vi "Scan Module.vi"(7 "Slice pattern":T1={"repitition"=14, "thick slice (um)"=500.0, "thin slice (um)"=100.0} {"thin slice (um)" format="%#_13g"; "thick slice (um)" format="%#_13g"}, 8 "Error In":errorcluster, 9 "System Parameters":T2={"Vibratome"={"Z Bottom [mm]"=0.0, "Pre Cut Dwell [s]"=1.0, "Blade Frequency [RPM]"=3000, "Slice Speed [mm/s]"=0.1, "Post Cut Dwell [s]"=4.0, "Ramp Time [s]"=0.5, "Start X [mm]"=80.5, "Start Y [mm]"=72.0, "Slice Length [mm]"=15.0, "Slice Axis"=enum."X Axis", "Controller VISA Ref"="COM3"}, "Table Stages"={"X Stage"={"Position"=0.0, "Is.Enabled?"=FALSE, "Is.Connected?"=FALSE, "Device SN"="45875688", "AccelerationMaximum"=50.0, "VelocityMaximum"=50.0, "Acceleration"=20.0, "Velocity"=20.0, "waitTimeout (ms)"=1000000, "Model"=enum."Thorlabs LTS", "Is.Homed?"=FALSE}, "Y Stage"={"Position"=0.0, "Is.Enabled?"=FALSE, "Is.Connected?"=FALSE, "Device SN"="45875512", "AccelerationMaximum"=50.0, "VelocityMaximum"=50.0, "Acceleration"=20.0, "Velocity"=20.0, "waitTimeout (ms)"=1000000, "Model"=enum."Thorlabs LTS", "Is.Homed?"=FALSE}, "Z Stage"={"Position"=0.0, "Is.Enabled?"=FALSE, "Is.Connected?"=FALSE, "Device SN"="49872414", "AccelerationMaximum"=50.0, "VelocityMaximum"=50.0, "Acceleration"=20.0, "Velocity"=20.0, "waitTimeout (ms)"=100000, "Model"=enum."Thorlabs MLJ", "Is.Homed?"=FALSE}}}, 10 "Mosaic Parameters":T5={"Overlap Options"={"Overlap Type"=enum."No Overlap", "Percent Overlap"=0, "Justify"=enum."Start"}, "Mosaic Range"={"X Axis"={"Start [mm]"=10.0, "Steps [pts]"=0, "End [mm]"=28.0}, "Y Axis"={"Start [mm]"=45.0, "Steps [pts]"=0, "End [mm]"=63.0}}, "Scan Pattern"=enum."Uni-directional", "Number of slices"=1} {"Overlap Options"."Percent Overlap" max=50}, 11 "Imaging Parameters":T6={"Save Path"=path "E:/Jiarui/1217test", "# Cscan"=1, "ROI Parameters"={"ROI (mm)"={"X (mm)"=1.0, "Y (mm)"=1.0}, "Shift (mm)"={"Xshift (mm)"=0.0, "Yshift (mm)"=0.0}}, "Scan Parameters"={"# Scan"={"#Ascan"=400, "#Bscan"=400}, "# Rpt"={"#ARpt"=1, "#BRpt"=1}, "Aline Rate"=2, "# Extra"={"# ARpt_extra"=5, "#Brtn_extra"=80}}, "Objective"=0, "Image Index"=0} {"Objective" items=["5X LKM05", "10X LKM10", "20X LKM20", "10X LSM02"]; "Scan Parameters"."Aline Rate" items=["76 KHz", "146 KHz", "76 KHz", "28 KHz", "10 KHz"]}) -> (0 "Error Out":errorcluster, 3 "Finished?":bool)   [LabVIEW 2017]
uses:
  Controls/Go Scan Actions.ctl
  Controls/System Parameters.ctl
  Hardware/Table Stage/Controls/Translation Stage Cluster.ctl
  Controls/Translation Stage Types.ctl
  Controls/FGV Actions.ctl
  Controls/ScanType.ctl
  Hardware/Table Stage/Controls/Motion Translation Module Control.ctl
  Controls/Set Get Controls.ctl
panel:
  out "Waveform Chart":dbl(graph)
  out "Current State":T7
  out "Current Position":cluster{"X":dbl, "Y":dbl}
  out "XY Graph":cluster{"X":dbl, "Y":dbl}[](graph)
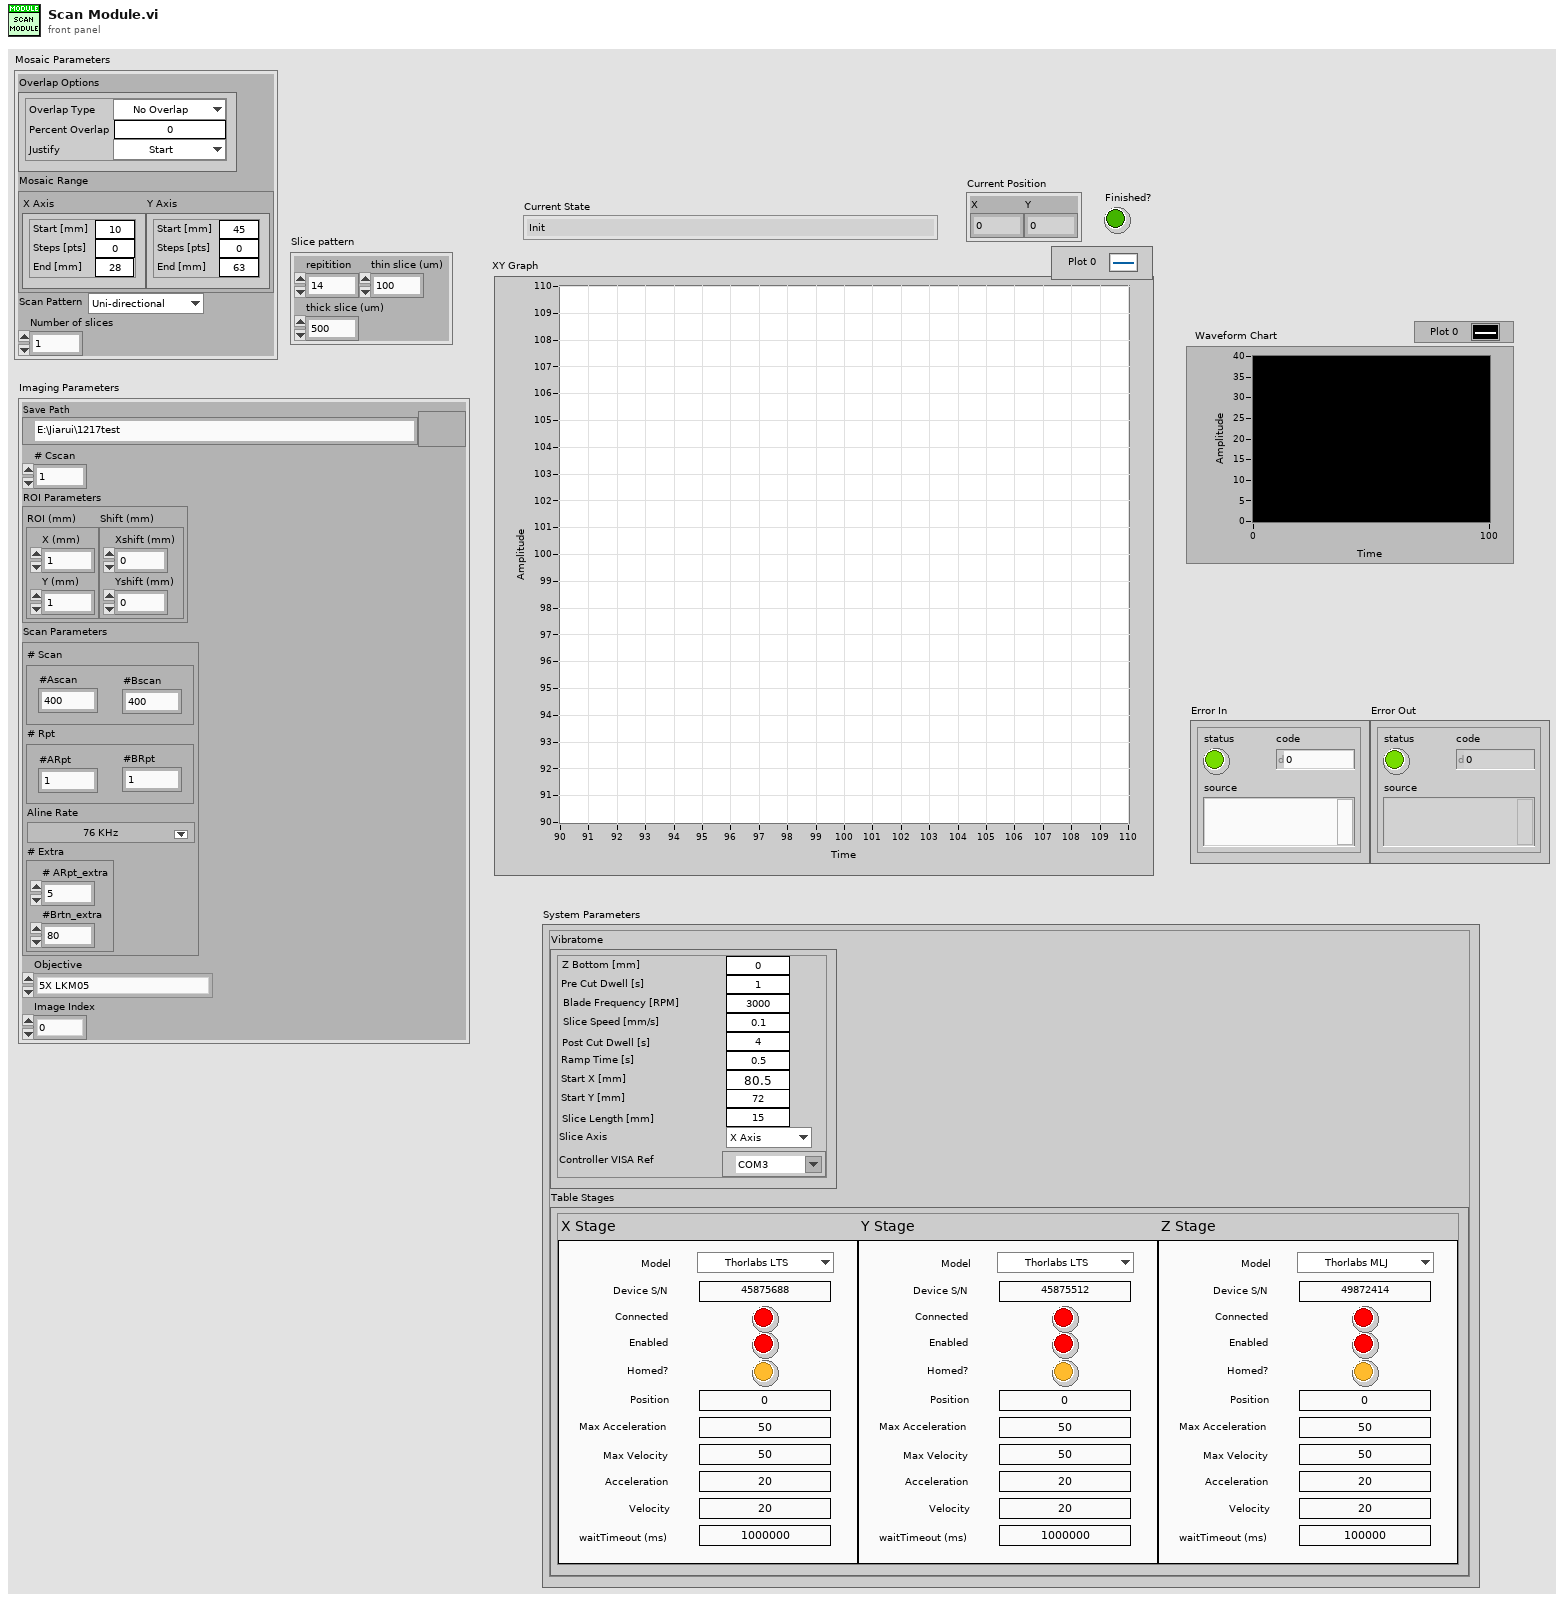
[diagram p1: front panel]
types:
  T1 = cluster{"repitition":i32, "thick slice (um)":dbl, "thin slice (um)":dbl}
  T2 = typedef "System Parameters.ctl" = cluster{"Vibratome":cluster{"Z Bottom [mm]":dbl, "Pre Cut Dwell [s]":dbl, "Blade Frequency [RPM]":u16, "Slice Speed [mm/s]":dbl, "Post Cut Dwell [s]":dbl, "Ramp Time [s]":dbl, "Start X [mm]":dbl, "Start Y [mm]":dbl, "Slice Length [mm]":dbl, "Slice Axis":enum16{"X Axis", "Y Axis", "Z Axis"}, "Controller VISA Ref":refnum<visa-resource-name>}, "Table Stages":cluster{"X Stage":T3, "Y Stage":T3, "Z Stage":T3}}
  T3 = typedef "Translation Stage Cluster.ctl" = cluster{"Position":dbl, "Is.Enabled?":bool, "Is.Connected?":bool, "Device SN":string, "AccelerationMaximum":dbl, "VelocityMaximum":dbl, "Acceleration":dbl, "Velocity":dbl, "waitTimeout (ms)":i32, "Model":T4, "Is.Homed?":bool}
  T4 = typedef "Translation Stage Types.ctl" = enum16{"None", "Thorlabs LTS", "Thorlabs MLJ"}
  T5 = cluster{"Overlap Options":cluster{"Overlap Type":enum16{"No Overlap", "X Only", "Y Only", "X and Y"}, "Percent Overlap":u8, "Justify":enum16{"Start", "Center", "End"}}, "Mosaic Range":cluster{"X Axis":cluster{"Start [mm]":dbl, "Steps [pts]":u16, "End [mm]":dbl}, "Y Axis":cluster{"Start [mm]":dbl, "Steps [pts]":u16, "End [mm]":dbl}}, "Scan Pattern":enum16{"Uni-directional", "Bi-Directional", "Spiral Out", "Spiral In"}, "Number of slices":i16}
  T6 = cluster{"Save Path":path, "# Cscan":i32, "ROI Parameters":cluster{"ROI (mm)":cluster{"X (mm)":sgl, "Y (mm)":sgl}, "Shift (mm)":cluster{"Xshift (mm)":sgl, "Yshift (mm)":sgl}}, "Scan Parameters":cluster{"# Scan":cluster{"#Ascan":i32, "#Bscan":i32}, "# Rpt":cluster{"#ARpt":i32, "#BRpt":i32}, "Aline Rate":u16, "# Extra":cluster{"# ARpt_extra":i32, "#Brtn_extra":i32}}, "Objective":u16, "Image Index":i16}
  T7 = typedef "Go Scan Actions.ctl" = enum16{"Init", "Init Scan Head", "Init Table Stage", "Init Vibratome", "Generate Mosaic", "Go Image Home", "Go Mosaic", "Acquire Image", "Go Vibratome", "Slice", "Finished"}
  T8 = cluster{"Start [mm]":dbl, "Steps [pts]":u16, "End [mm]":dbl}
  T9 = enum16{"Uni-directional", "Bi-Directional", "Spiral Out", "Spiral In"}
  T10 = cluster{"Overlap Type":enum16{"No Overlap", "X Only", "Y Only", "X and Y"}, "Percent Overlap":u8, "Justify":enum16{"Start", "Center", "End"}}
  T11 = typedef "FGV Actions.ctl" = enum16{"Init", "Set", "Get", "Clear"}
  T12 = typedef "ScanType.ctl" = enum16{"Single Frame", "Continuous Frame", "ROI Line", "Vibratome", "Mosaic", "Mosaic + Slice"}
  T13 = enum16{"Init", "Configure", "Configure Data", "Generate Scan Pattern", "Start Acquire Raw", "Start Acquire Data", "Acquire RAW", "Acquire Data", "Stop Acquire", "Uninit"}
  T14 = enum16{"Create", "Enqueue", "Dequeue", "Release"}
  T15 = typedef "Set Get Controls.ctl" = enum16{"Set", "Get"}
  T16 = typedef "Motion Translation Module Control.ctl" = enum16{"Init", "Home", "Status", "Velocity/Accel", "Position", "Jog", "Stop", "Uninit", "Enable", "Disable"}
  T17 = cluster{"Objective":u16, "Aline Rate":u16, "# Cscan":i32, "ROI Parameters":cluster{"ROI (mm)":cluster{"X (mm)":sgl, "Y (mm)":sgl}, "Shift (mm)":cluster{"Xshift (mm)":sgl, "Yshift (mm)":sgl}}}
  T18 = cluster{"Image Index":i16, "Slice Index":i16, "#Cscan":i32, "nAT per B":i32, "nA per B":i32, "Brtn_extra/2":i32}
  T19 = cluster{"# Scan":cluster{"#Ascan":i32, "#Bscan":i32}, "# Rpt":cluster{"#ARpt":i32, "#BRpt":i32}, "Aline Rate":u16, "# Extra":cluster{"# ARpt_extra":i32, "#Brtn_extra":i32}}
  T20 = cluster{"ROI (mm)":cluster{"X (mm)":sgl, "Y (mm)":sgl}, "Shift (mm)":cluster{"Xshift (mm)":sgl, "Yshift (mm)":sgl}}
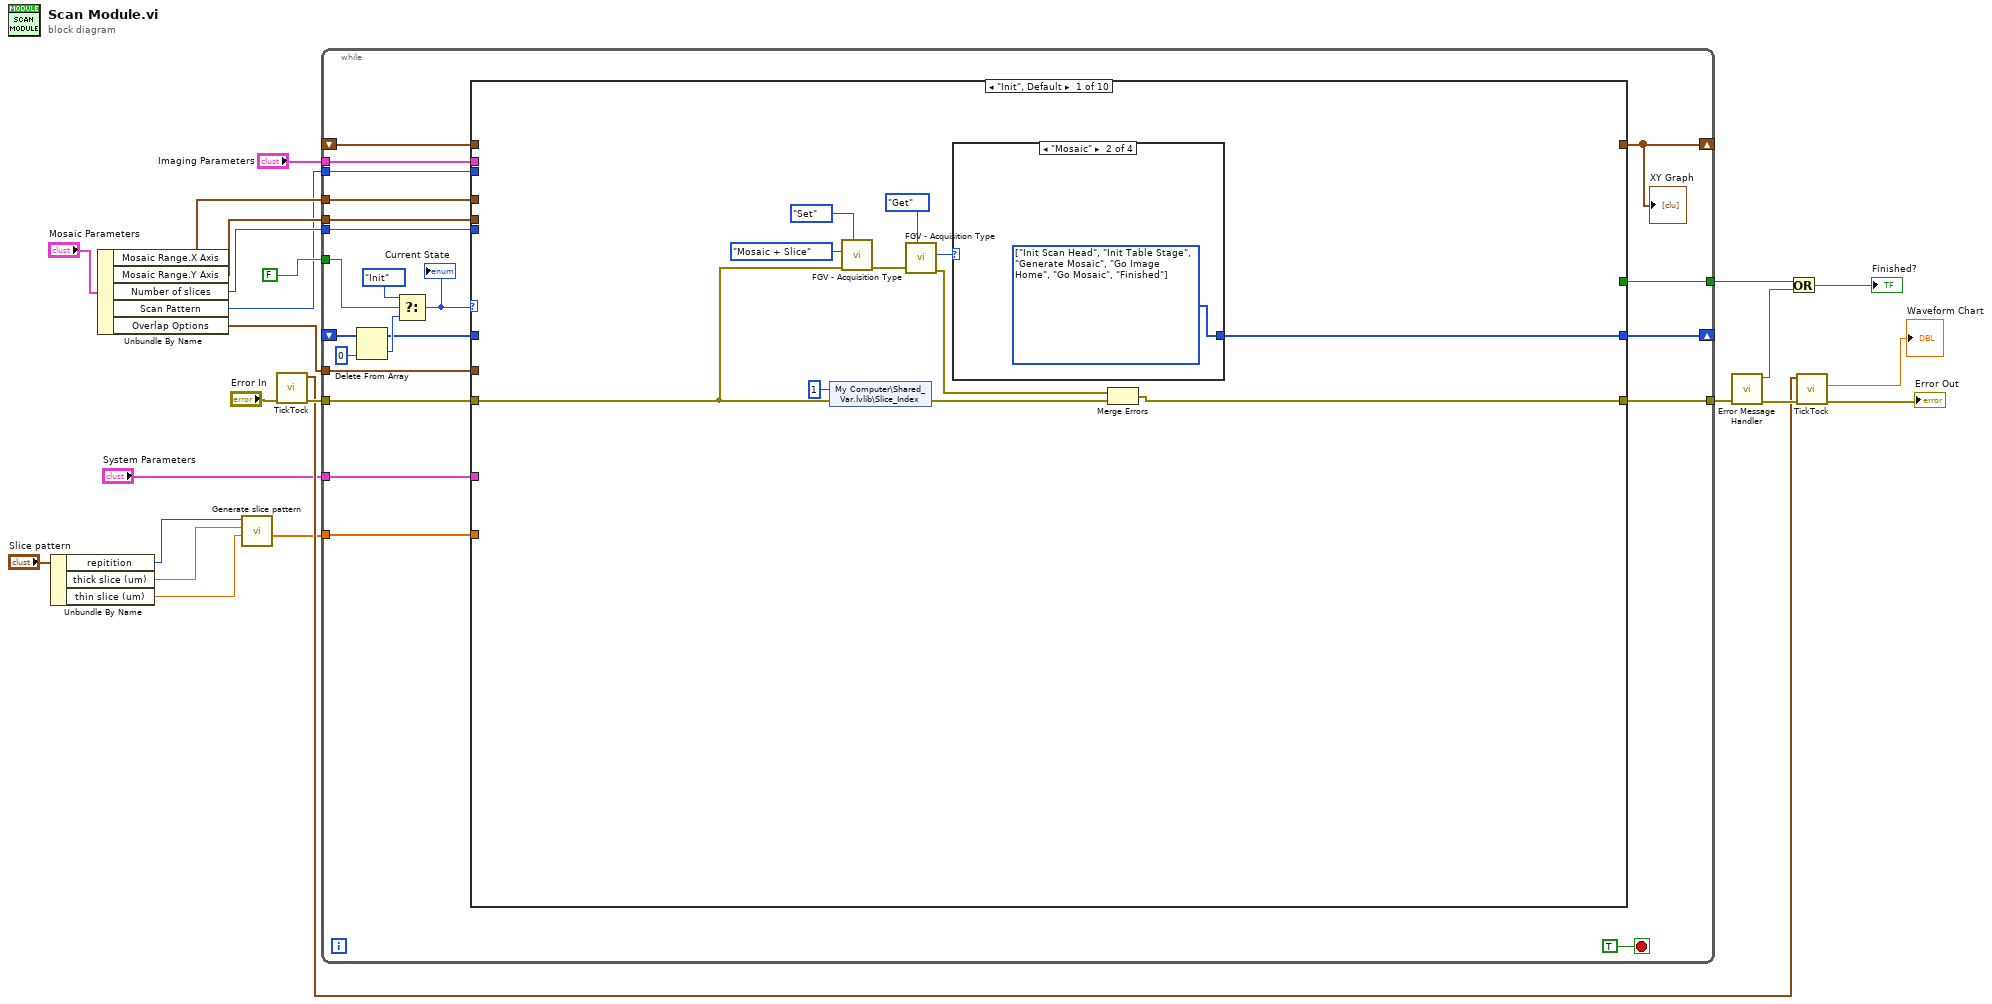
[diagram p0: block diagram]
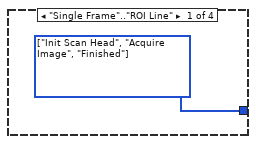
[diagram p2: hidden frame]
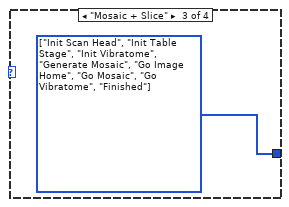
[diagram p3: hidden frame]
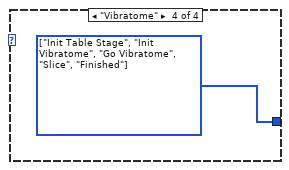
[diagram p4: hidden frame]
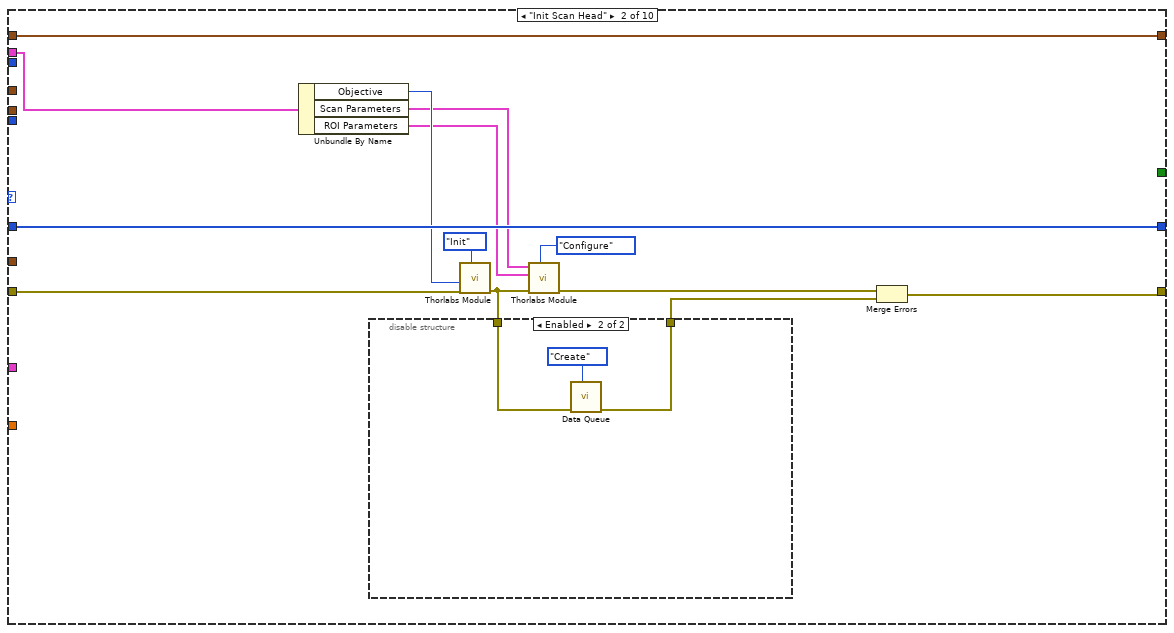
[diagram p5: hidden frame]
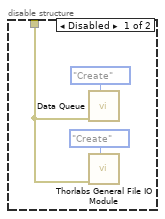
[diagram p6: hidden frame]
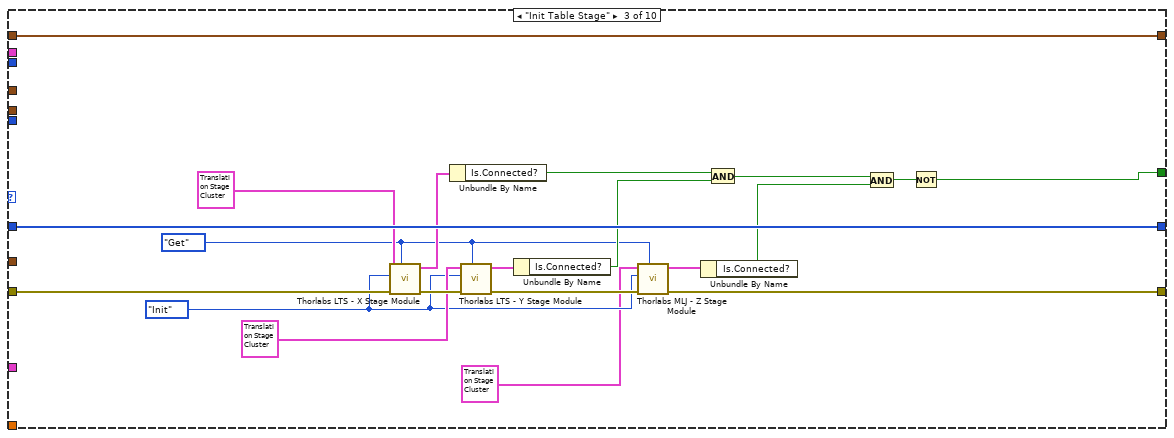
[diagram p7: hidden frame]
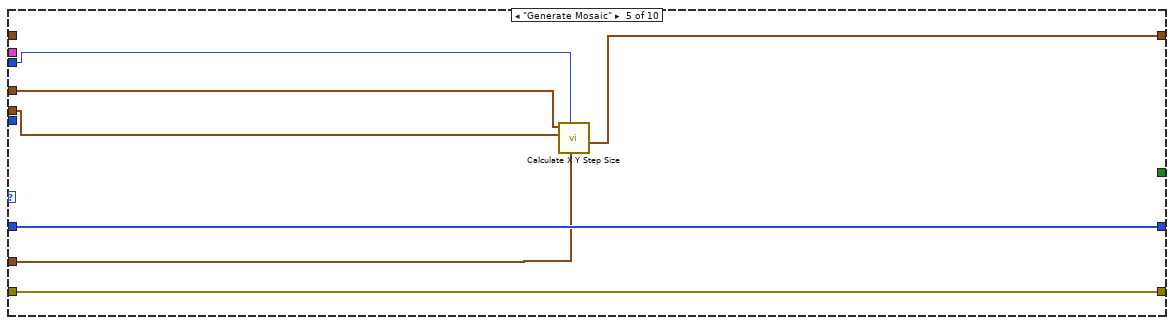
[diagram p9: hidden frame]
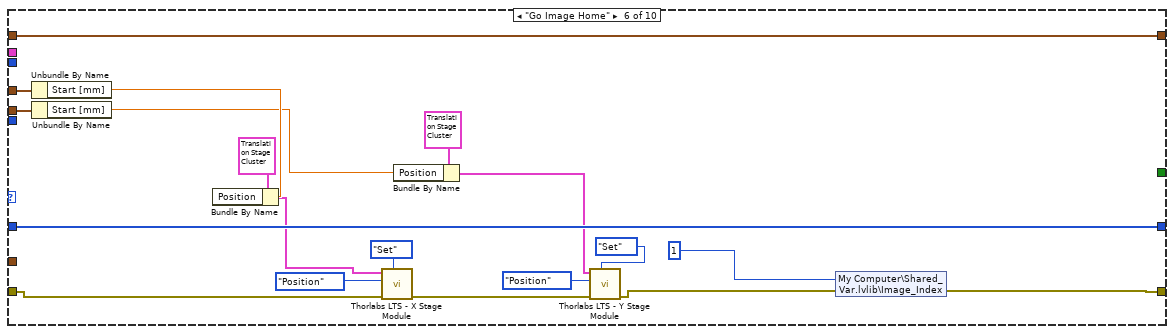
[diagram p10: hidden frame]
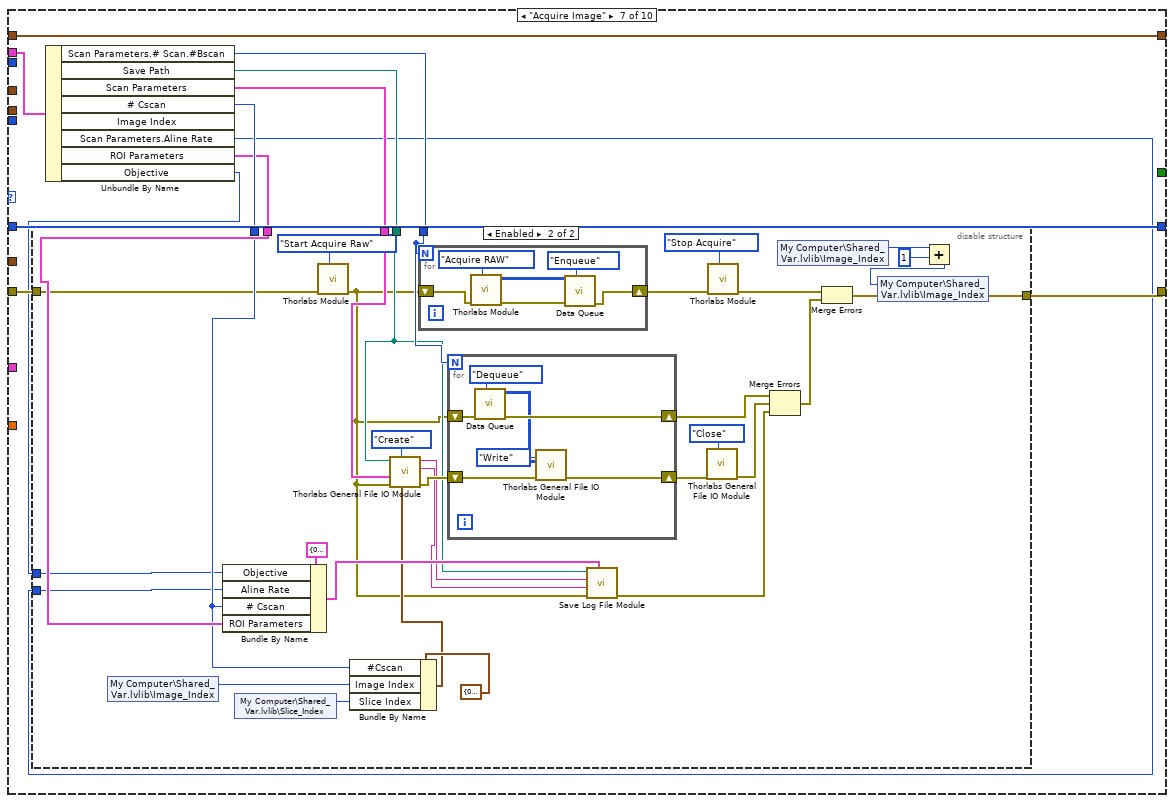
[diagram p11: hidden frame]
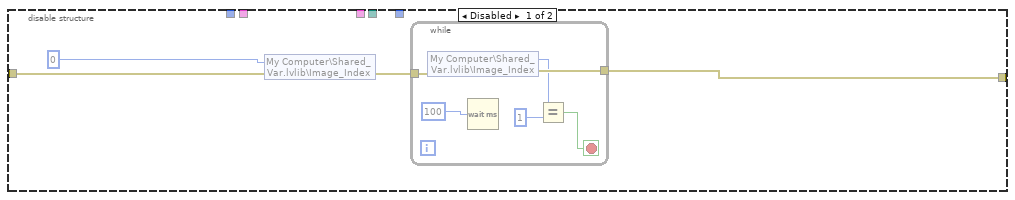
[diagram p12: hidden frame]
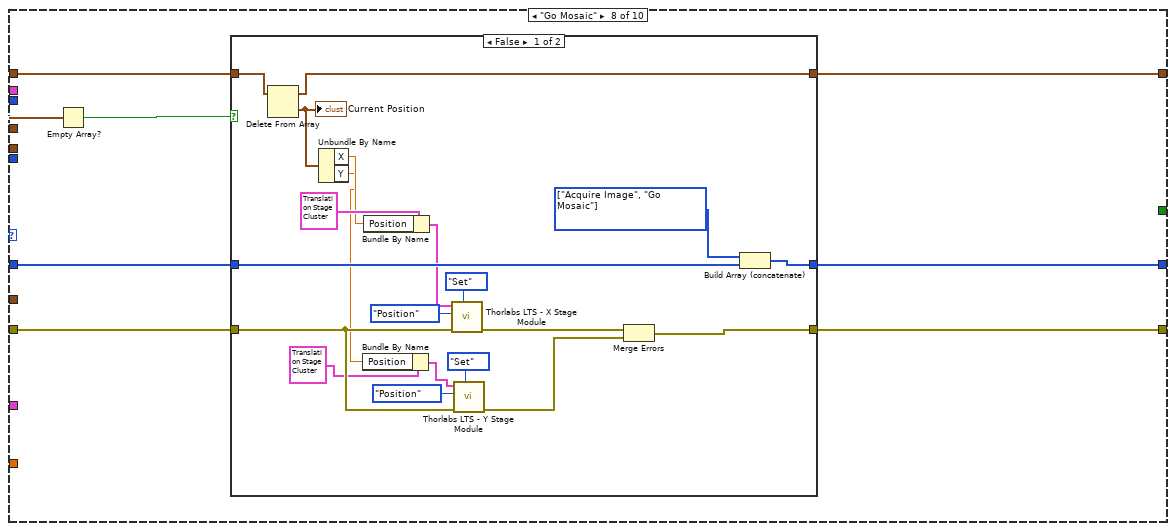
[diagram p13: hidden frame]
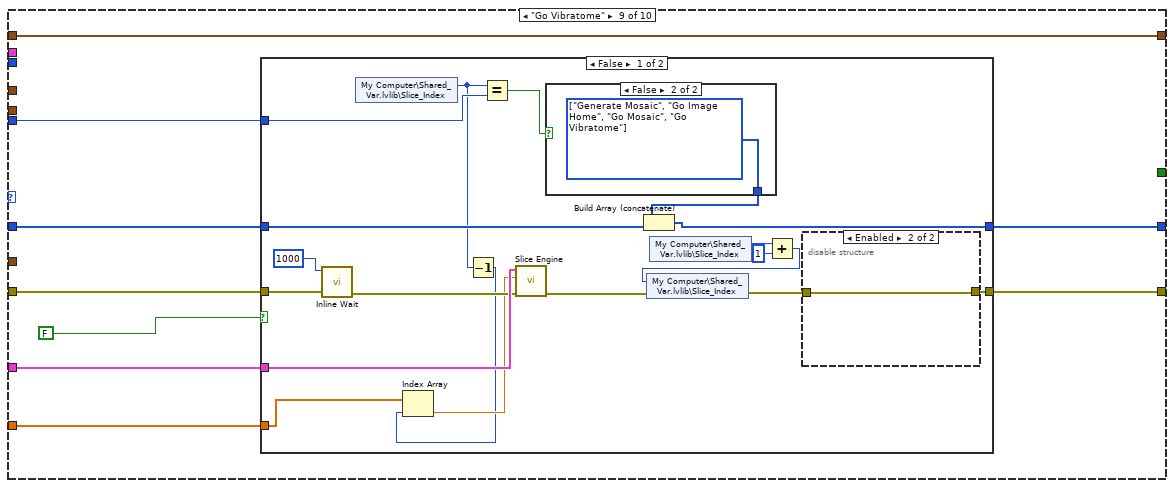
[diagram p15: hidden frame]
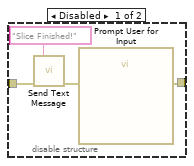
[diagram p16: hidden frame]
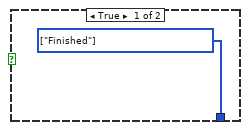
[diagram p17: hidden frame]
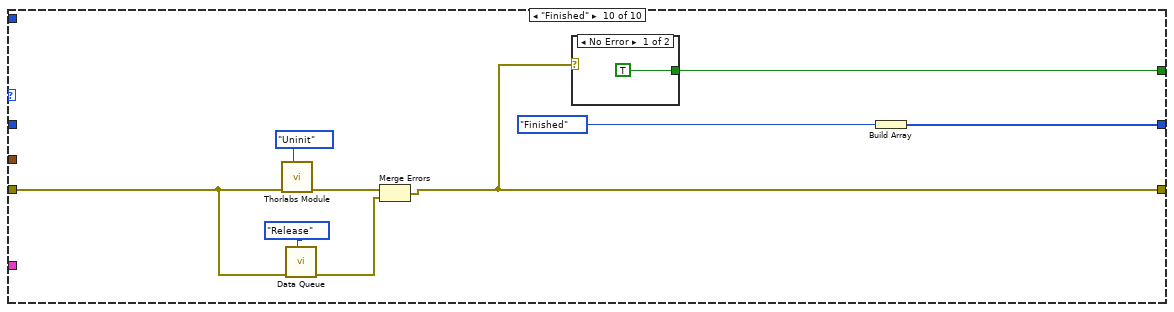
[diagram p19: hidden frame]
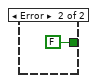
[diagram p20: hidden frame]
diagram:
  n1 = Unbundle By Name("Slice pattern") -> ("repitition"=w3:i32, "thick slice (um)"=w2:dbl, "thin slice (um)"=w1:dbl)
  n2 = Unbundle By Name("Mosaic Parameters") -> ("Mosaic Range.X Axis"=w12:T8, "Mosaic Range.Y Axis"=w11:T8, "Number of slices"=w9:i16, "Scan Pattern"=w7:T9, "Overlap Options"=w8:T10)
  n3 = call "Generate slice pattern.vi"("thin slice (um)"=w1, "thick slice (um)"=w2, "repitition"=w3) -> ("Array"=w5:dbl[])  [unwired: 8 in]
  n4 = call "TickTock.vi"("Error In"="Error In") -> ("Error Out"=w17:errorcluster, "Current Time (Out)"=w15:timestamp)  [unwired: 8 in, 1 out]
  n5 = while {
    shift-right: [w43] -> _
    shift-left: _ -> [w42]
    tunnel: FALSE ("Init") -> [w45]
    shift-right: [w38] -> _
    shift-left: _ -> [w39]
    tunnel: [w37] -> w23
    tunnel: w17 -> [w35]
    tunnel: [w34] -> w22
    tunnel: w12 -> [w32]
    tunnel: w11 -> [w31]
    tunnel: "Imaging Parameters" -> [w30]
    tunnel: w9 -> [w29]
    tunnel: w8 -> [w28]
    tunnel: w7 -> [w27]
    tunnel: "System Parameters" -> [w26]
    tunnel: w5 -> [w25]
    stop <- TRUE stop-if-true
    n6 = Delete From Array(array=w42, index=0) -> (deleted portion=w41:T7, array with subset deleted=w40:T7[])  [unwired: 1 in]
    n7 = Select(t=Go_Scan_Actions."Init", s=w45, f=w41) -> (s? t:f=w44:T7)
    "Current State" <- w44
    n8 = case shown="\"Init\", Default" w44 {
      tunnel: [w55 w73 w99 w102 w110 w128 w140 w201 w234 w273] -> w43
      tunnel: w40 -> [_ w73 w99 w102 w110 w128 w140 w202 w235 _]
      tunnel: [_ w74 w100 w103 w108 w129 w141 w205 w237 _] -> w38
      tunnel: w39 -> [_ w74 w100 w103 _ w129 w141 w204 w237 _]
      tunnel: [_ _ w94 _ _ _ _ _ _ w272] -> w37
      tunnel: w35 -> [w49 w71 w98 w101 w109 w124 w139 w200 w233 w271]
      tunnel: [w50 w64 w88 w101 w109 w127 w138 w199 w232 w266] -> w34
      tunnel: w32 -> [_ _ _ _ w107 w125 _ _ _ _]
      tunnel: w31 -> [_ _ _ _ w106 w115 _ _ _ _]
      tunnel: w30 -> [_ w72 _ _ _ _ w137 _ _ _]
      tunnel: w29 -> [_ _ _ _ _ _ _ _ w231 _]
      tunnel: w28 -> [_ _ _ _ w105 _ _ _ _ _]
      tunnel: w27 -> [_ _ _ _ w104 _ _ _ _ _]
      tunnel: w26 -> [_ _ _ _ _ _ _ _ w230 _]
      tunnel: w25 -> [_ _ _ _ _ _ _ _ w229 _]
      frame "Init", Default {
        n9 = shared-variable "My Computer\\Shared_Var.lvlib\\Slice_Index"(i16 1 ("Image_Index"), error in=w49) -> (error out=w52:errorcluster)
        n10 = call "FGV - Acquisition Type.vi"("Actions"=FGV_Actions."Set", "Error In"=w49, "Scan Type [In]"=ScanType."Mosaic + Slice") -> ("Error Out"=w53:errorcluster)  [unwired: 6 in, 2 out]
        n11 = call "FGV - Acquisition Type.vi"("Actions"=FGV_Actions."Get", "Error In"=w53) -> ("Error Out"=w51:errorcluster, "Scan Type [Out]"=w56:T12)  [unwired: 7 in, 1 out]
        n12 = case shown="\"Mosaic\"" w56 {
          tunnel: [w58 w59 w60 w61] -> w55
          frame "Single Frame".."ROI Line" {
            w58 = T7[] [enum."Init Scan Head", enum."Acquire Image", enum."Finished"] items=["Init", "Init Scan Head", "Init Table Stage", "Init Vibratome", "Generate Mosaic", "Go Image Home", "Go Mosaic", "Acquire Image", "Go Vibratome", "Slice", "Finished"]
          }
          frame "Mosaic" {
            w59 = T7[] [enum."Init Scan Head", enum."Init Table Stage", enum."Generate Mosaic", enum."Go Image Home", enum."Go Mosaic", enum."Finished"] items=["Init", "Init Scan Head", "Init Table Stage", "Init Vibratome", "Generate Mosaic", "Go Image Home", "Go Mosaic", "Acquire Image", "Go Vibratome", "Slice", "Finished"]
          }
          frame "Mosaic + Slice" {
            w60 = T7[] [enum."Init Scan Head", enum."Init Table Stage", enum."Init Vibratome", enum."Generate Mosaic", enum."Go Image Home", enum."Go Mosaic", enum."Go Vibratome", enum."Finished"] items=["Init", "Init Scan Head", "Init Table Stage", "Init Vibratome", "Generate Mosaic", "Go Image Home", "Go Mosaic", "Acquire Image", "Go Vibratome", "Slice", "Finished"]
          }
          frame "Vibratome" {
            w61 = T7[] [enum."Init Table Stage", enum."Init Vibratome", enum."Go Vibratome", enum."Slice", enum."Finished"] items=["Init", "Init Scan Head", "Init Table Stage", "Init Vibratome", "Generate Mosaic", "Go Image Home", "Go Mosaic", "Acquire Image", "Go Vibratome", "Slice", "Finished"]
          }
        }
        n13 = Merge Errors(w51, w52) -> (w50:errorcluster)
      }
      frame "Init Scan Head" {
        n14 = Unbundle By Name(w72) -> ("Objective"=w70:u16, "Scan Parameters"=w69:T19, "ROI Parameters"=w68:T20)
        n15 = call "Thorlabs Module.vi"("Actions"=T13."Init", "error in"=w71, "Objective"=w70) -> ("error out"=w67:errorcluster)  [unwired: 6 in, 2 out]
        n16 = disable-structure shown="Enabled" {
          disable-tunnel: w67 -> [w75 w79]
          disable-tunnel: [_ w78] -> w65
          frame Disabled {
            n17 = call "Data Queue.vi"("Action"=T14."Create", "error in (no error)"=w75) -> ()  [unwired: 8 in, 2 out]
            n18 = call "Thorlabs General File IO Module.vi"("Actions"=enum16{"Create", "Write", "Close"}."Create", "error in"=w75) -> ()  [unwired: 7 in, 3 out]
          }
          frame Enabled {
            n19 = call "Data Queue.vi"("Action"=T14."Create", "error in (no error)"=w79) -> ("error out"=w78:errorcluster)  [unwired: 8 in, 1 out]
          }
        }
        n20 = call "Thorlabs Module.vi"("Actions"=T13."Configure", "error in"=w67, "ROI Parameters"=w68, "Scan Parameters"=w69) -> ("error out"=w66:errorcluster)  [unwired: 5 in, 2 out]
        n21 = Merge Errors(w66, w65) -> (w64:errorcluster)
      }
      frame "Init Table Stage" {
        w87 = Set_Get_Controls."Get" ("Set/Get")
        w86 = Motion_Translation_Module_Control."Init" ("Action")
        n22 = call "Thorlabs LTS - X Stage Module.vi"("Set/Get"=w87, "Error In"=w98, "Action"=w86, "Cluster In"=T3 {"Position"=0.0, "Is.Enabled?"=TRUE, "Is.Connected?"=FALSE, "Device SN"="45876060", "AccelerationMaximum"=0.0, "VelocityMaximum"=0.0, "Acceleration"=0.0, "Velocity"=0.0, "waitTimeout (ms)"=10000000, "Model"=enum."Thorlabs LTS", "Is.Homed?"=FALSE}) -> ("Error Out"=w97:errorcluster, "Cluster Out"=w96:T3)  [unwired: 6 in]
        n23 = Unbundle By Name(w96) -> ("Is.Connected?"=w95:bool)
        n24 = call "Thorlabs LTS - Y Stage Module.vi"("Set/Get"=w87, "Error In"=w97, "Action"=w86, "Cluster In"=T3 {"Position"=0.0, "Is.Enabled?"=TRUE, "Is.Connected?"=FALSE, "Device SN"="45875512", "AccelerationMaximum"=0.0, "VelocityMaximum"=0.0, "Acceleration"=0.0, "Velocity"=0.0, "waitTimeout (ms)"=1000000, "Model"=enum."Thorlabs LTS", "Is.Homed?"=FALSE}) -> ("Error Out"=w89:errorcluster, "Cluster Out"=w91:T3)  [unwired: 6 in]
        n25 = Unbundle By Name(w91) -> ("Is.Connected?"=w90:bool)
        n26 = call "Thorlabs MLJ - Z Stage Module.vi"("Set/Get"=w87, "Error In"=w89, "Action"=w86, "Cluster In"=T3 {"Position"=0.0, "Is.Enabled?"=TRUE, "Is.Connected?"=FALSE, "Device SN"="49872414", "AccelerationMaximum"=0.0, "VelocityMaximum"=0.0, "Acceleration"=0.0, "Velocity"=0.0, "waitTimeout (ms)"=1000000, "Model"=enum."Thorlabs MLJ", "Is.Homed?"=FALSE}) -> ("Error Out"=w88:errorcluster, "Cluster Out"=w84:T3)  [unwired: 6 in]
        n27 = Unbundle By Name(w84) -> ("Is.Connected?"=w83:bool)
        n28 = And(x=w95, y=w90) -> (x .and. y?=w82:bool)
        n29 = And(x=w82, y=w83) -> (x .and. y?=w81:bool)
        n30 = Not(x=w81) -> (.not. x?=w94:bool)
      }
      frame "Init Vibratome" {
      }
      frame "Generate Mosaic" {
        n31 = call "Calculate X Y Step Size.vi"("Overlap Options"=w105, "Scan Pattern"=w104, "Y Axis"=w106, "X Axis"=w107) -> ("Array"=w108:cluster{"X":dbl, "Y":dbl}[])  [unwired: 4 in, 3 out]
      }
      frame "Go Image Home" {
        n32 = Unbundle By Name(w125) -> ("Start [mm]"=w120:dbl)
        n33 = Unbundle By Name(w115) -> ("Start [mm]"=w114:dbl)
        n34 = Bundle By Name(cluster=T3 {"Position"=0.0, "Is.Enabled?"=FALSE, "Is.Connected?"=FALSE, "Device SN"="45876060", "AccelerationMaximum"=0.0, "VelocityMaximum"=0.0, "Acceleration"=0.0, "Velocity"=0.0, "waitTimeout (ms)"=10000000, "Model"=enum."Thorlabs LTS", "Is.Homed?"=FALSE} ("Cluster In"), "Position"=w120) -> (w119:T3)
        n35 = call "Thorlabs LTS - X Stage Module.vi"("Set/Get"=Set_Get_Controls."Set", "Error In"=w124, "Action"=Motion_Translation_Module_Control."Position", "Cluster In"=w119) -> ("Error Out"=w113:errorcluster)  [unwired: 6 in, 1 out]
        n36 = Bundle By Name(cluster=T3 {"Position"=0.0, "Is.Enabled?"=FALSE, "Is.Connected?"=FALSE, "Device SN"="45875512", "AccelerationMaximum"=0.0, "VelocityMaximum"=0.0, "Acceleration"=0.0, "Velocity"=0.0, "waitTimeout (ms)"=10000000, "Model"=enum."Thorlabs LTS", "Is.Homed?"=FALSE} ("Cluster In"), "Position"=w114) -> (w118:T3)
        n37 = call "Thorlabs LTS - Y Stage Module.vi"("Set/Get"=Set_Get_Controls."Set", "Error In"=w113, "Action"=Motion_Translation_Module_Control."Position", "Cluster In"=w118) -> ("Error Out"=w112:errorcluster)  [unwired: 6 in, 1 out]
        n38 = shared-variable "My Computer\\Shared_Var.lvlib\\Image_Index"(i16 1 ("Image_Index"), error in=w112) -> (error out=w127:errorcluster)
      }
      frame "Acquire Image" {
        n39 = Unbundle By Name(w137) -> ("Scan Parameters.# Scan.#Bscan"=w136:i32, "Save Path"=w135:path, "Scan Parameters"=w134:T19, "# Cscan"=w133:i32, "Scan Parameters.Aline Rate"=w131:u16, "ROI Parameters"=w132:T20, "Objective"=w130:u16)  [unwired: 1 out]
        n40 = disable-structure shown="Enabled" {
          disable-tunnel: w139 -> [w144 w152]
          disable-tunnel: [w142 w174] -> w138
          disable-tunnel: w136 -> [_ w178]
          disable-tunnel: w135 -> [_ w161]
          disable-tunnel: w134 -> [_ w159]
          disable-tunnel: w133 -> [_ w181]
          disable-tunnel: w132 -> [_ w182]
          disable-tunnel: w131 -> [_ w180]
          disable-tunnel: w130 -> [_ w179]
          frame Disabled {
            n41 = shared-variable "My Computer\\Shared_Var.lvlib\\Image_Index"(i16 0 ("Image_Status"), error in=w144) -> (error out=w143:errorcluster)
            n42 = while {
              tunnel: w143 -> [w150]
              tunnel: [w149] -> w142
              stop <- w148 stop-if-true
              n43 = shared-variable "My Computer\\Shared_Var.lvlib\\Image_Index"(error in=w150) -> (w147:i16, error out=w149:errorcluster)
              n44 = Wait (ms)(milliseconds to wait=u32 100) -> ()  [unwired: 1 out]
              n45 = Equal?(x=w147, y=i16 1) -> (x = y?=w148:bool)
            }
          }
          frame Enabled {
            n46 = shared-variable "My Computer\\Shared_Var.lvlib\\Image_Index"() -> (w165:i16)  [unwired: 1 in, 1 out]
            n47 = Bundle By Name(cluster=T17 {"Objective"=0, "Aline Rate"=2, "# Cscan"=1, "ROI Parameters"={"ROI (mm)"={"X (mm)"=1.0, "Y (mm)"=1.0}, "Shift (mm)"={"Xshift (mm)"=0.0, "Yshift (mm)"=0.0}}} ("Log Header Parameters"), "Objective"=w179, "Aline Rate"=w180, "# Cscan"=w181, "ROI Parameters"=w182) -> (w166:T17)
            n48 = shared-variable "My Computer\\Shared_Var.lvlib\\Slice_Index"() -> (w169:i16)  [unwired: 1 in, 1 out]
            n49 = call "Thorlabs Module.vi"("Actions"=T13."Start Acquire Raw", "error in"=w152) -> ("error out"=w158:errorcluster)  [unwired: 7 in, 2 out]
            n50 = Bundle By Name(cluster=T18 {"Image Index"=0, "Slice Index"=0, "#Cscan"=0, "nAT per B"=0, "nA per B"=0, "Brtn_extra/2"=0} ("input cluster"), "#Cscan"=w181, "Image Index"=w165, "Slice Index"=w169) -> (w160:T18)
            n51 = call "Thorlabs General File IO Module.vi"("Imaging Parameters"=w160, "Actions"=enum16{"Create", "Write", "Write Data", "Close"}."Create", "error in"=w158, "Scan Parameters"=w159, "Save Path"=w161) -> ("error out"=w164:errorcluster, "Scan Parameter"=w162:string, "Save Name"=w163:string)  [unwired: 4 in]
            n52 = for {
              N: w178 -> [_]
              shift-right: [w195] -> w184
              shift-left: w158 -> [w198]
              n53 = call "Thorlabs Module.vi"("Actions"=T13."Acquire RAW", "error in"=w198) -> ("error out"=w196:errorcluster, "Raw Data Out"=w193:u16[][])  [unwired: 7 in, 1 out]
              n54 = call "Data Queue.vi"("Action"=T14."Enqueue", "error in (no error)"=w196, "Data In"=w193) -> ("error out"=w195:errorcluster)  [unwired: 7 in, 1 out]
            }
            n55 = for {
              N: w178 -> [_]
              shift-right: [w191] -> w157
              shift-left: w158 -> [w190]
              shift-right: [w189] -> w171
              shift-left: w164 -> [w188]
              n56 = call "Data Queue.vi"("Action"=T14."Dequeue", "error in (no error)"=w190) -> ("error out"=w191:errorcluster, "Data Out"=w186:u16[][])  [unwired: 8 in]
              n57 = call "Thorlabs General File IO Module.vi"("Actions"=enum16{"Create", "Write", "Write Data", "Close"}."Write", "error in"=w188, "Raw Data In"=w186) -> ("error out"=w189:errorcluster)  [unwired: 6 in, 2 out]
            }
            n58 = call "Save Log File Module.vi"("Log Header Parameters"=w166, "error in (no error)"=w158, "Scan Parameter"=w162, "Save Name"=w163, "Save Path"=w161) -> ("error out"=w170:errorcluster)  [unwired: 6 in]
            n59 = call "Thorlabs General File IO Module.vi"("Actions"=enum16{"Create", "Write", "Write Data", "Close"}."Close", "error in"=w171) -> ("error out"=w172:errorcluster)  [unwired: 7 in, 2 out]
            n60 = call "Thorlabs Module.vi"("Actions"=T13."Stop Acquire", "error in"=w184) -> ("error out"=w183:errorcluster)  [unwired: 7 in, 2 out]
            n61 = Merge Errors(w157, w172, w170) -> (w185:errorcluster)
            n62 = shared-variable "My Computer\\Shared_Var.lvlib\\Image_Index"() -> (w177:i16)  [unwired: 1 in, 1 out]
            n63 = Merge Errors(w183, w185) -> (w175:errorcluster)
            n64 = Add(x=w177, y=i16 1) -> (x+y=w173:i16)
            n65 = shared-variable "My Computer\\Shared_Var.lvlib\\Image_Index"(w173, error in=w175) -> (error out=w174:errorcluster)
          }
        }
      }
      frame "Go Mosaic" {
        n66 = Empty Array?(array=w204) -> (empty?=w203:bool)
        n67 = case shown="False" w203 {
          tunnel: [w225 w228] -> w205
          tunnel: w204 -> [w224 w228]
          tunnel: w202 -> [w223 w227]
          tunnel: [w221 w227] -> w201
          tunnel: w200 -> [w211 w226]
          tunnel: [w207 w226] -> w199
          frame False {
            w220 = T7[] [enum."Acquire Image", enum."Go Mosaic"] items=["Init", "Init Scan Head", "Init Table Stage", "Init Vibratome", "Generate Mosaic", "Go Image Home", "Go Mosaic", "Acquire Image", "Go Vibratome", "Slice", "Finished"]
            n68 = Delete From Array(array=w224) -> (deleted portion=w222:cluster{"X":dbl, "Y":dbl}, array with subset deleted=w225:cluster{"X":dbl, "Y":dbl}[])  [unwired: 2 in]
            "Current Position" <- w222
            n69 = Unbundle By Name(w222) -> ("X"=w215:dbl, "Y"=w209:dbl)
            n70 = Bundle By Name(cluster=T3 {"Position"=0.0, "Is.Enabled?"=FALSE, "Is.Connected?"=FALSE, "Device SN"="45875512", "AccelerationMaximum"=0.0, "VelocityMaximum"=0.0, "Acceleration"=0.0, "Velocity"=0.0, "waitTimeout (ms)"=10000000, "Model"=enum."None", "Is.Homed?"=FALSE} ("Cluster In"), "Position"=w209) -> (w208:T3)
            n71 = Bundle By Name(cluster=T3 {"Position"=0.0, "Is.Enabled?"=FALSE, "Is.Connected?"=FALSE, "Device SN"="45875688", "AccelerationMaximum"=0.0, "VelocityMaximum"=0.0, "Acceleration"=0.0, "Velocity"=0.0, "waitTimeout (ms)"=10000000, "Model"=enum."None", "Is.Homed?"=FALSE} ("Cluster In"), "Position"=w215) -> (w214:T3)
            n72 = call "Thorlabs LTS - X Stage Module.vi"("Set/Get"=Set_Get_Controls."Set", "Error In"=w211, "Action"=Motion_Translation_Module_Control."Position", "Cluster In"=w214) -> ("Error Out"=w218:errorcluster)  [unwired: 6 in, 1 out]
            n73 = call "Thorlabs LTS - Y Stage Module.vi"("Set/Get"=Set_Get_Controls."Set", "Error In"=w211, "Action"=Motion_Translation_Module_Control."Position", "Cluster In"=w208) -> ("Error Out"=w206:errorcluster)  [unwired: 6 in, 1 out]
            n74 = Merge Errors(w218, w206) -> (w207:errorcluster)
            n75 = Build Array (concatenate)(w220, w223) -> (w221:T7[])
          }
          frame True {
          }
        }
      }
      frame "Go Vibratome" {
        n76 = case shown="False" FALSE ("No Slice?") {
          tunnel: w235 -> [w256 w265]
          tunnel: [w255 w265] -> w234
          tunnel: w233 -> [w249 w264]
          tunnel: [w242 w264] -> w232
          tunnel: w231 -> [w247 _]
          tunnel: w230 -> [w245 _]
          tunnel: w229 -> [w240 _]
          frame False {
            n77 = call "Inline Wait.vi"("Error In"=w249, "milliseconds to wait"=u32 1000) -> ("Error Out"=w244:errorcluster)  [unwired: 9 in]
            n78 = shared-variable "My Computer\\Shared_Var.lvlib\\Slice_Index"() -> (w239:i16)  [unwired: 1 in, 1 out]
            n79 = Decrement(x=w239) -> (x-1=w238:i16)
            n80 = Index Array(array=w240, index=w238) -> (element=w241:dbl)
            n81 = Equal?(x=w239, y=w247) -> (x = y?=w250:bool)
            n82 = call "Slice Engine.vi"("error in (no error)"=w244, "Slice thickness  (mm)"=w241, "System Parameters"=w245) -> ("error out"=w246:errorcluster)  [unwired: 8 in]
            n83 = case shown="False" w250 {
              tunnel: [w262 w263] -> w254
              frame True {
                w262 = T7[] [enum."Finished"] items=["Init", "Init Scan Head", "Init Table Stage", "Init Vibratome", "Generate Mosaic", "Go Image Home", "Go Mosaic", "Acquire Image", "Go Vibratome", "Slice", "Finished"]
              }
              frame False {
                w263 = T7[] [enum."Generate Mosaic", enum."Go Image Home", enum."Go Mosaic", enum."Go Vibratome"] items=["Init", "Init Scan Head", "Init Table Stage", "Init Vibratome", "Generate Mosaic", "Go Image Home", "Go Mosaic", "Acquire Image", "Go Vibratome", "Slice", "Finished"]
              }
            }
            n84 = Build Array (concatenate)(w254, w256) -> (w255:T7[])
            n85 = shared-variable "My Computer\\Shared_Var.lvlib\\Slice_Index"() -> (w253:i16)  [unwired: 1 in, 1 out]
            n86 = Add(x=w253, y=i16 1) -> (x+y=w251:i16)
            n87 = shared-variable "My Computer\\Shared_Var.lvlib\\Slice_Index"(w251, error in=w246) -> (error out=w243:errorcluster)
            n88 = disable-structure shown="Enabled" {
              disable-tunnel: w243 -> [w260 w261]
              disable-tunnel: [w259 w261] -> w242
              frame Disabled {
                n89 = call "Send Text Message.vi"("error in"=w260, "subject"="Slice Finished!") -> ("error out"=w258:errorcluster)  [unwired: 9 in]
                n90 = call "Prompt User for Input"("error in (no error)"=w258) -> ("error out"=w259:errorcluster)  [unwired: 17 in, 1 out]
              }
              frame Enabled {
              }
            }
          }
          frame True {
          }
        }
      }
      frame "Finished" {
        n91 = call "Thorlabs Module.vi"("Actions"=T13."Uninit", "error in"=w271) -> ("error out"=w269:errorcluster)  [unwired: 7 in, 2 out]
        n92 = call "Data Queue.vi"("Action"=T14."Release", "error in (no error)"=w271) -> ("error out"=w268:errorcluster)  [unwired: 8 in, 1 out]
        n93 = Merge Errors(w269, w268) -> (w266:errorcluster)
        n94 = case shown="No Error" w266 {
          tunnel: [TRUE FALSE] -> w272
          frame No Error {
          }
          frame Error {
          }
        }
        n95 = Build Array(Go_Scan_Actions."Finished") -> (w273:T7[])
      }
    }
    "XY Graph" <- w38
  }
  n96 = call "Error Message Handler.vi"("Error In"=w22) -> ("Error Out"=w21:errorcluster, "T button?"=w19:bool)  [unwired: 9 in]
  n97 = Or(x=w23, y=w19) -> (x .or. y?=→"Finished?":bool)
  n98 = call "TickTock.vi"("Error In"=w21, "Current Time (In)"=w15) -> ("Error Out"=→"Error Out":errorcluster, "dt"=→"Waveform Chart":dbl)  [unwired: 7 in, 1 out]
